vi "Page_Info_Validate_Filename.vi"(8 "error in (no error)":errorcluster, 10 "Filename in":string, 11 "AB_PackedLibrary in":refnum<class "AB_PackedLibrary.lvclass">) -> (0 "error out":errorcluster, 1 "hasInvalidCharacters":bool, 2 "Filename out":string, 3 "AB_PackedLibrary out":refnum<class "AB_PackedLibrary.lvclass">, 5 "message":string)   [LabVIEW 2020, in "AB_PackedLibrary.lvclass"]
uses:
  <vilib>/AppBuilder/AB_Classes/PackedLib/AB_PackedLibrary.lvclass
  <vilib>/AppBuilder/AB_Classes/TargetFile/AB_Targetfile.lvclass
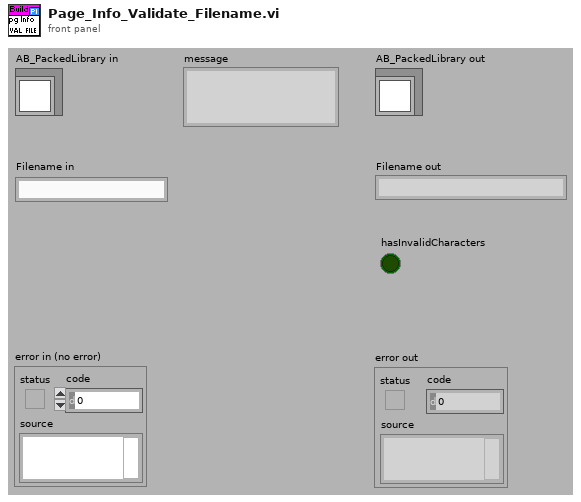
[diagram p1: front panel]
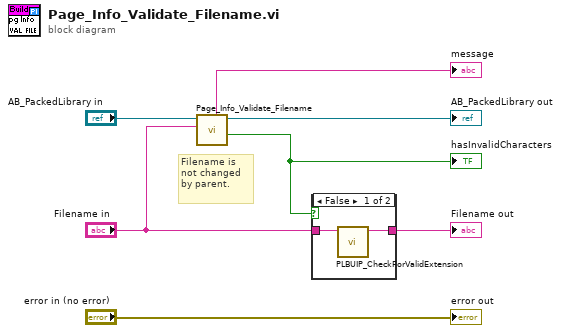
[diagram p0: block diagram]
diagram:
  # "Filename is not changed by parent."
  n1 = call-parent "Page_Info_Validate_Filename.vi"("Filename in"="Filename in", "AB_Targetfile in"="AB_PackedLibrary in") -> ("hasInvalidCharacters"=w4:bool, "AB_Targetfile out"=→"AB_PackedLibrary out":refnum<class "AB_PackedLibrary.lvclass">, "message"=→"message":string)  [unwired: 5 in, 2 out]
  "hasInvalidCharacters" <- w4
  n2 = case shown="False" w4 {
    tunnel: [w8 w10] -> w2
    tunnel: "Filename in" -> [w9 w10]
    frame False {
      n3 = call <resource>:"PLBUIP_CheckForValidExtension.vi"("Filename in"=w9) -> ("Filename out"=w8:string)  [unwired: 9 in, 1 out]
    }
    frame True {
    }
  }
  "Filename out" <- w2
  "error out" <- "error in (no error)"
